vi "test_graph_history.vi"() -> ()   [LabVIEW 2018]
panel:
  in  "pos":T1(graph)
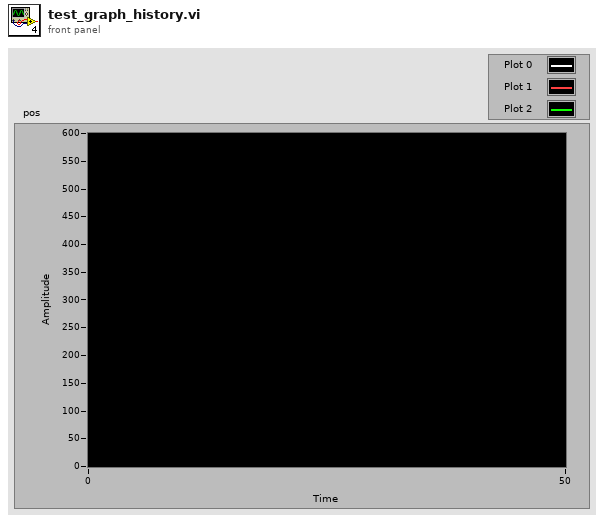
[diagram p1: front panel]
types:
  T1 = cluster{"Slide":i16, "set pt":i16, "position":i16}
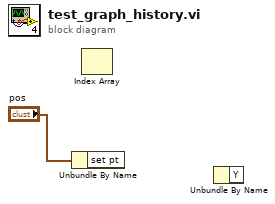
[diagram p0: block diagram]
diagram:
  n1 = Unbundle By Name("pos") -> ()  [unwired: 1 out]
  n2 = Index Array() -> ()  [unwired: 2 in, 1 out]
  n3 = Unbundle By Name() -> ()  [unwired: 1 in, 1 out]
